vi "ErrorXYZsearcher.vi"(8 "error Y":errorcluster, 10 "error Z":errorcluster, 11 "error X":errorcluster) -> (0 "error out":errorcluster)   [LabVIEW 2014]
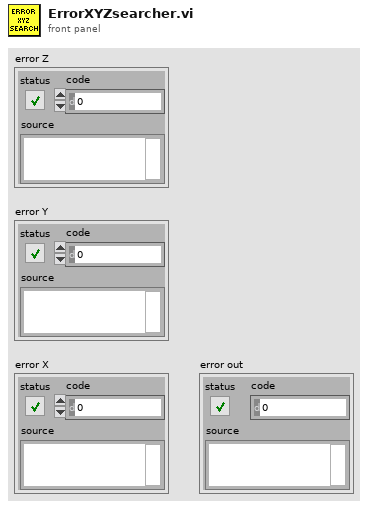
[diagram p1: front panel]
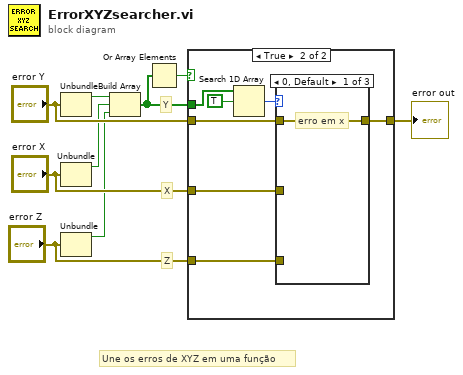
[diagram p0: block diagram]
diagram:
  # "Une os erros de XYZ em uma função"
  # "Z"
  # "Y"
  # "X"
  n1 = Unbundle("error Y") -> ("status"=w1:bool)  [unwired: 2 out]
  n2 = Unbundle("error X") -> ("status"=w2:bool)  [unwired: 2 out]
  n3 = Unbundle("error Z") -> ("status"=w3:bool)  [unwired: 2 out]
  n4 = Build Array(w1, w2, w3) -> (w6:bool[])
  n5 = Or Array Elements(Boolean array=w6) -> (logical OR=w4:bool)
  n6 = case shown="True" w4 {
    tunnel: "error Y" -> [w10 w14]
    tunnel: [w10 w13] -> w9
    tunnel: w6 -> [_ w17]
    tunnel: "error X" -> [_ w12]
    tunnel: "error Z" -> [_ w11]
    frame False {
    }
    frame True {
      n7 = Search 1D Array(1D array=w17, element=TRUE) -> (index of element=w15:i32)  [unwired: 1 in]
      n8 = case shown="0, Default" w15 {
        tunnel: w14 -> [w18 _ _]
        tunnel: [w18 w19 w20] -> w13
        tunnel: w12 -> [_ _ w20]
        tunnel: w11 -> [_ w19 _]
        frame 0, Default {
          # "erro em x"
        }
        frame 2 {
          # "erro em z"
        }
        frame 1 {
          # "erro em y"
        }
      }
    }
  }
  "error out" <- w9
